vi "Add-parameter-tab-elements.vi"(8 "error in (no error)":errorcluster, 11 "Controls in":refnum<vi>[](array[refnum])) -> (0 "error out":errorcluster, 3 "Controls out":refnum<vi>[](array[refnum]))   [LabVIEW 2013, in "CameraVision.lvlib" / "CV-UI.lvclass"]
uses:
  CV-UI.lvclass
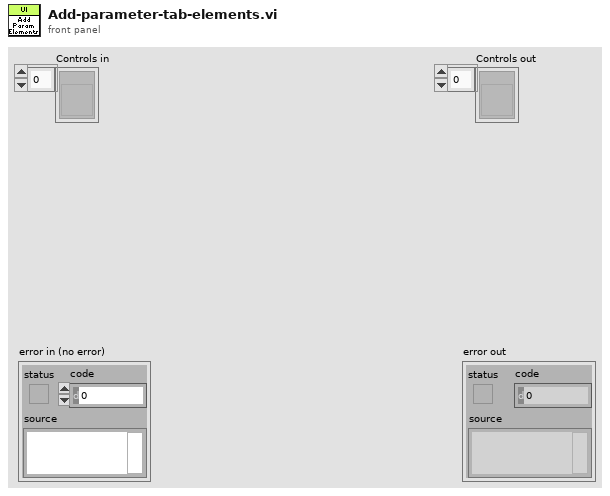
[diagram p1: front panel]
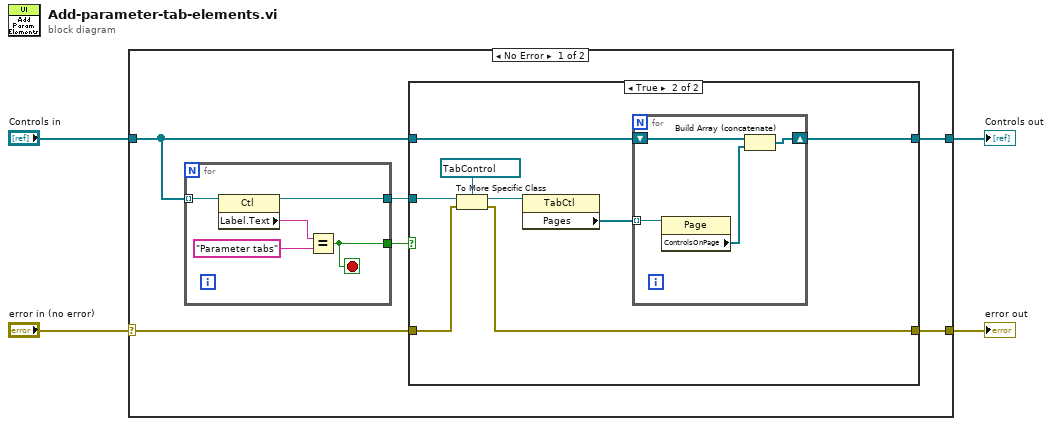
[diagram p0: block diagram]
diagram:
  n1 = case shown="No Error" "error in (no error)" {
    selector: "error in (no error)" -> [w10 w31]
    tunnel: [w5 w31] -> w3
    tunnel: "Controls in" -> [w9 w30]
    tunnel: [w6 w30] -> w1
    frame No Error {
      n2 = for {
        tunnel: w9 -> [w29] mode=indexing
        tunnel: [w26] -> w8
        tunnel: [w25] -> w7
        stop <- w26 stop-if-true
        n3 = property class="Ctl"(reference=w29) -> (reference out=w25:refnum<vi>, "Label.Text"=w28:string)  [unwired: 1 in, 1 out]
        n4 = Equal?(x=w28, y="Parameter tabs") -> (x = y?=w26:bool)
      }
      n5 = case shown="True" w8 {
        tunnel: w10 -> [w11 w17]
        tunnel: w9 -> [w12 w15]
        tunnel: w7 -> [_ w18]
        tunnel: [w12 w14] -> w6
        tunnel: [w11 w13] -> w5
        frame False {
        }
        frame True {
          n6 = To More Specific Class(target class=refnum<vi> refnum ("Motor tabs"), reference=w18, error in=w17) -> (specific class reference=w19:refnum<vi>, error out=w13:errorcluster)
          n7 = property class="TabCtl"(reference=w19) -> ("Pages"=w16:refnum<vi>[])  [unwired: 1 in, 2 out]
          n8 = for {
            tunnel: w16 -> [w24] mode=indexing
            shift-right: [w21] -> w14
            shift-left: w15 -> [w23]
            n9 = property class="Page"(reference=w24) -> ("ControlsOnPage"=w22:refnum<vi>[])  [unwired: 1 in, 2 out]
            n10 = Build Array (concatenate)(w23, w22) -> (w21:refnum<vi>[])
          }
        }
      }
    }
    frame Error {
    }
  }
  "error out" <- w3
  "Controls out" <- w1
